vi "Parameters_Build_Reference.vi"(10 "Reference Move Parameters":T1={"Reference Move Mode"=3, "Start Search Forward"=FALSE, "Stop on FWD Edge"=FALSE, "Approach Forward"=FALSE, "Velocity"=0.0, "Acceleration"=0.0}, 11 "Axis to command":i32) -> (3 "Parameters":dbl[](array[numeric]))   [LabVIEW 2017, in "WordManipulationLibrary.lvlib"]
uses:
  WordManipulationLibrary.lvlib
  Parameters_Reference.ctl
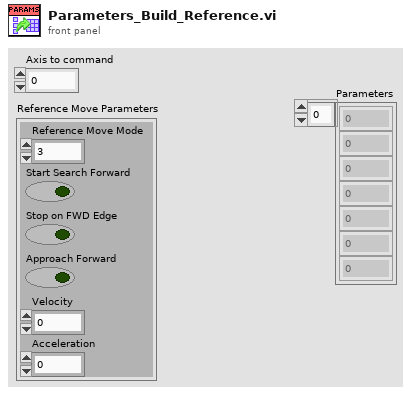
[diagram p1: front panel]
types:
  T1 = typedef "WordManipulationLibrary.lvlib/Parameters_Reference.ctl" = cluster{"Reference Move Mode":i32, "Start Search Forward":bool, "Stop on FWD Edge":bool, "Approach Forward":bool, "Velocity":dbl, "Acceleration":dbl}
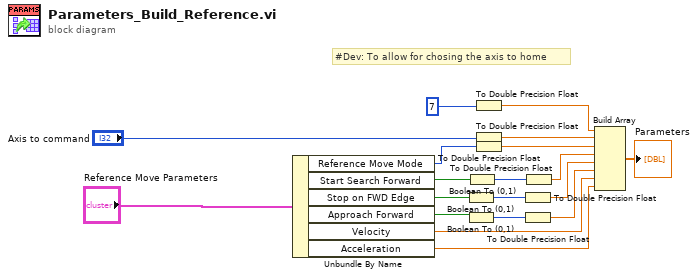
[diagram p0: block diagram]
diagram:
  # "#Dev: To allow for chosing the axis to home"
  n1 = Unbundle By Name("Reference Move Parameters") -> ("Reference Move Mode"=w10:i32, "Start Search Forward"=w17:bool, "Stop on FWD Edge"=w13:bool, "Approach Forward"=w12:bool, "Velocity"=w6:dbl, "Acceleration"=w5:dbl)
  n2 = Boolean To (0,1)(Boolean=w13) -> (0, 1=w15:i16)
  n3 = Boolean To (0,1)(Boolean=w12) -> (0, 1=w14:i16)
  n4 = Boolean To (0,1)(Boolean=w17) -> (0, 1=w16:i16)
  n5 = To Double Precision Float(number=i16 7 ("element")) -> (double precision float=w1:dbl)
  n6 = To Double Precision Float(number="Axis to command") -> (double precision float=w3:dbl)
  n7 = To Double Precision Float(number=w10) -> (double precision float=w18:dbl)
  n8 = To Double Precision Float(number=w15) -> (double precision float=w8:dbl)
  n9 = To Double Precision Float(number=w14) -> (double precision float=w7:dbl)
  n10 = To Double Precision Float(number=w16) -> (double precision float=w9:dbl)
  n11 = Build Array(w1, w3, w18, w9, w8, w7, w6, w5) -> (→"Parameters":dbl[])
